vi "Git_Push.vi"(8 "error in (no error)":errorcluster caption="entrée d'erreur (pas d'erreur)", 9 "Branch Name":string, 10 "Remote Name":string, 11 "Chemin in":path) -> (0 "error out":errorcluster caption="sortie d'erreur", 3 "Chemin out":path)   [LabVIEW 2021]
uses:
  <userlib>/_OpenG.lib/file/file.llb/File Exists - Scalar__ogtk.vi
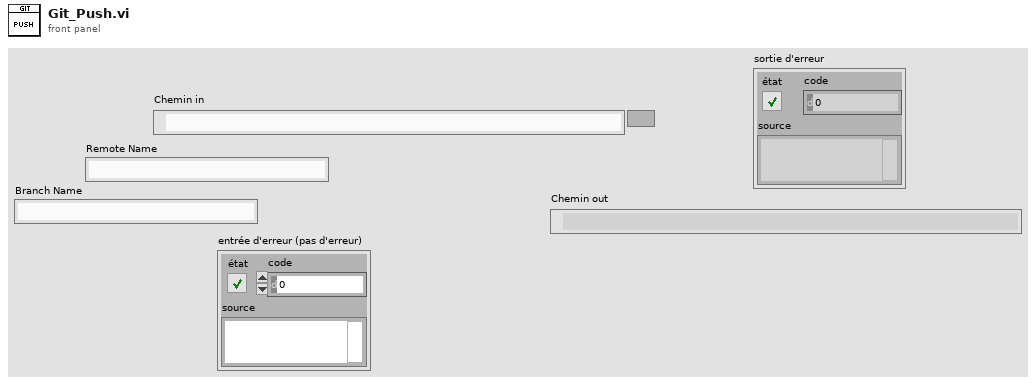
[diagram p1: front panel]
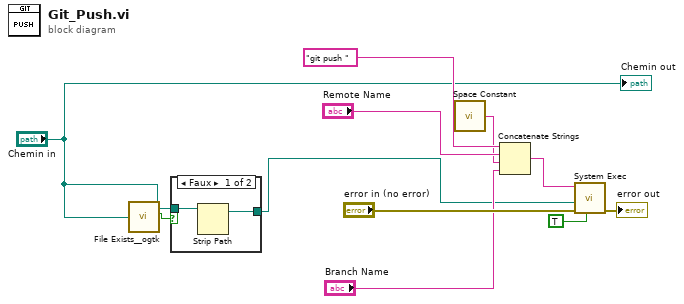
[diagram p0: block diagram]
diagram:
  n1 = call-poly <userlib>:"File Exists__ogtk.vi"("file path"="Chemin in") -> ("is directory"=w3:bool)  [unwired: 6 in, 1 out]
  n2 = case shown="Faux" w3 {
    tunnel: [w13 w14] -> w1
    tunnel: "Chemin in" -> [w12 w14]
    frame False {
      n3 = Strip Path(path=w12) -> (stripped path=w13:path)  [unwired: 1 out]
    }
    frame True {
    }
  }
  n4 = call <vilib>:"Space Constant.vi"() -> ("String"=w5:string)
  n5 = Concatenate Strings("git push ", "Remote Name", w5, "Branch Name") -> (w10:string)
  n6 = call <vilib>:"System Exec.vi"("run minimized? (F)"=TRUE, "error in (no error)"="error in (no error)", "working directory"=w1, "command line"=w10) -> ("error out"=→"error out":errorcluster)  [unwired: 4 in, 3 out]
  "Chemin out" <- "Chemin in"
